vi "Offset Locking- Main v1.0.vi"() -> ()   [LabVIEW 2017]
uses:
  <vilib>/Utility/error.llb/DialogType.ctl
  <vilib>/measure/mamon.llb/Waveform Peak Detection for 1 Chan.vi
  <vilib>/addons/control/pid/pid.llb/PID Advanced (DBL).vi
  <vilib>/measure/NI_MAPro.lvlib
  <vilib>/addons/control/pid/NI_PID_pid.lvlib
  <vilib>/Analysis/NI_AALBase.lvlib
panel:
  out "Run Time (min)":dbl
  out "standard deviation":dbl format="%0.3e"
  in  "Ref Peak 2":i32=1
  in  "Ref Peak":i32=2
  in  "First Cal Peak":i32
  in  "Last Cal Peak":i32=2
  out "# found":i32
  out "Offset":dbl(graph)
  in  "Manual PZT Control":dbl format="%#_g V"
  in  "Engage PZT PID?":bool
  out "Offset (GHz)":dbl format="%#_4g"
  in  "# of Shots for Averaging":i32=100
  in  "Name Convention":string="Chirp Offset Lock Log"
  in  "Save Directory":path=path "C:/Users/LabUser/Google Drive/Measurements/04-2018"
  out "Four peaks?":bool
  out "PID Output":dbl(graph)
  in  "PID Gains":T1={"proportional gain (Kc)"=-1.0, "integral time (Ti, min)"=0.01, "derivative time (Td, min)"=0.0} {"derivative time (Td, min)" format="%.3f"; "integral time (Ti, min)" format="%.3f"; "proportional gain (Kc)" format="%.3f"}
  in  "Setpoint Range (GHz)":cluster{"setpoint high":dbl, "setpoint low":dbl}={"setpoint high"=7.7901, "setpoint low"=7.7899} {"setpoint high" format="%.4f"; "setpoint low" format="%.4f"}
  out "dt out (s)":dbl format="%.3f"
  in  "Frequency Offset Setpoint (GHz)":dbl=7.79 format="%.3f"
  out "GHz/sec":dbl
  out "dt":dbl format="%#_4g"
  out "Locations":dbl[](array[numeric]) format="%.2p"
  out "Amplitudes":dbl[](array[numeric]) format="%.2p"
  out "2nd Derivatives":dbl[](array[numeric]) format="%.2p"
  out "10 GHz FPI":dynamicdata(graph)
  in  "Stop":bool
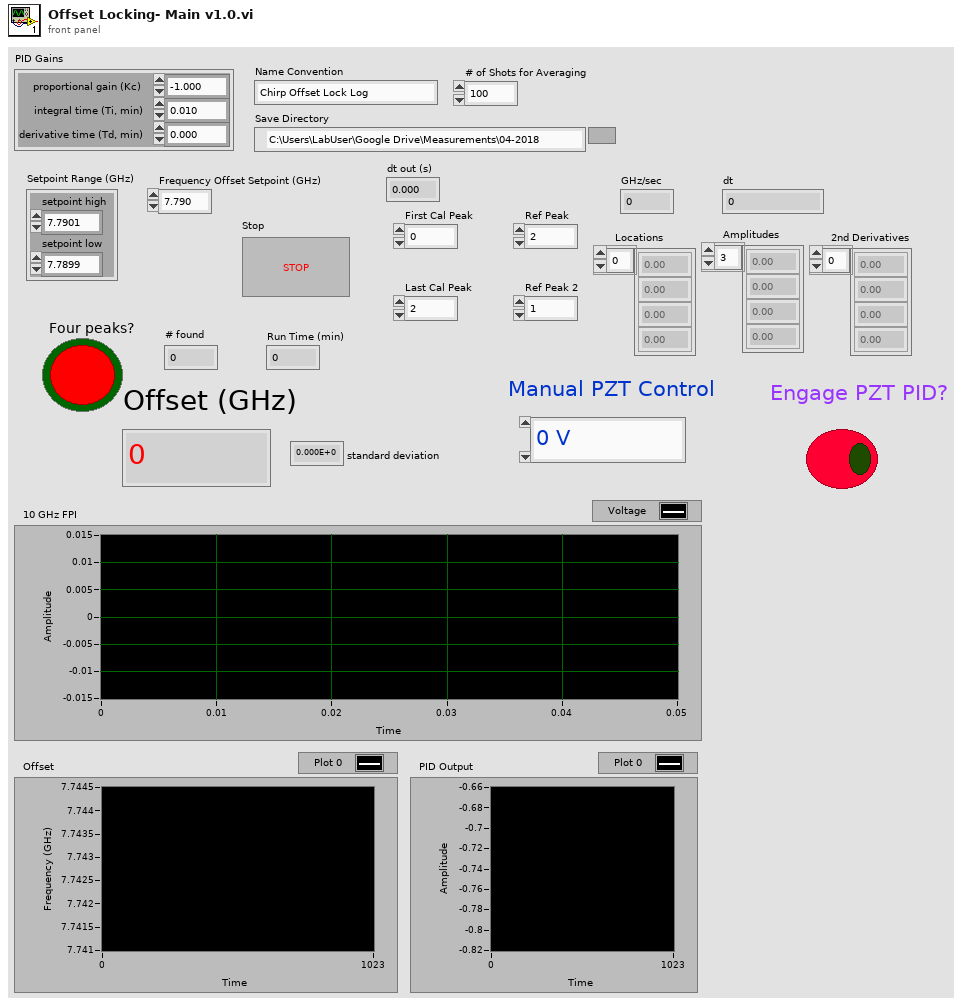
[diagram p1: front panel]
types:
  T1 = cluster{"proportional gain (Kc)":dbl, "integral time (Ti, min)":dbl, "derivative time (Td, min)":dbl}
  T2 = enum8{"Enabled", "Disabled", "Disabled and Grayed Out"}
  T3 = typedef "DialogType.ctl" = u16
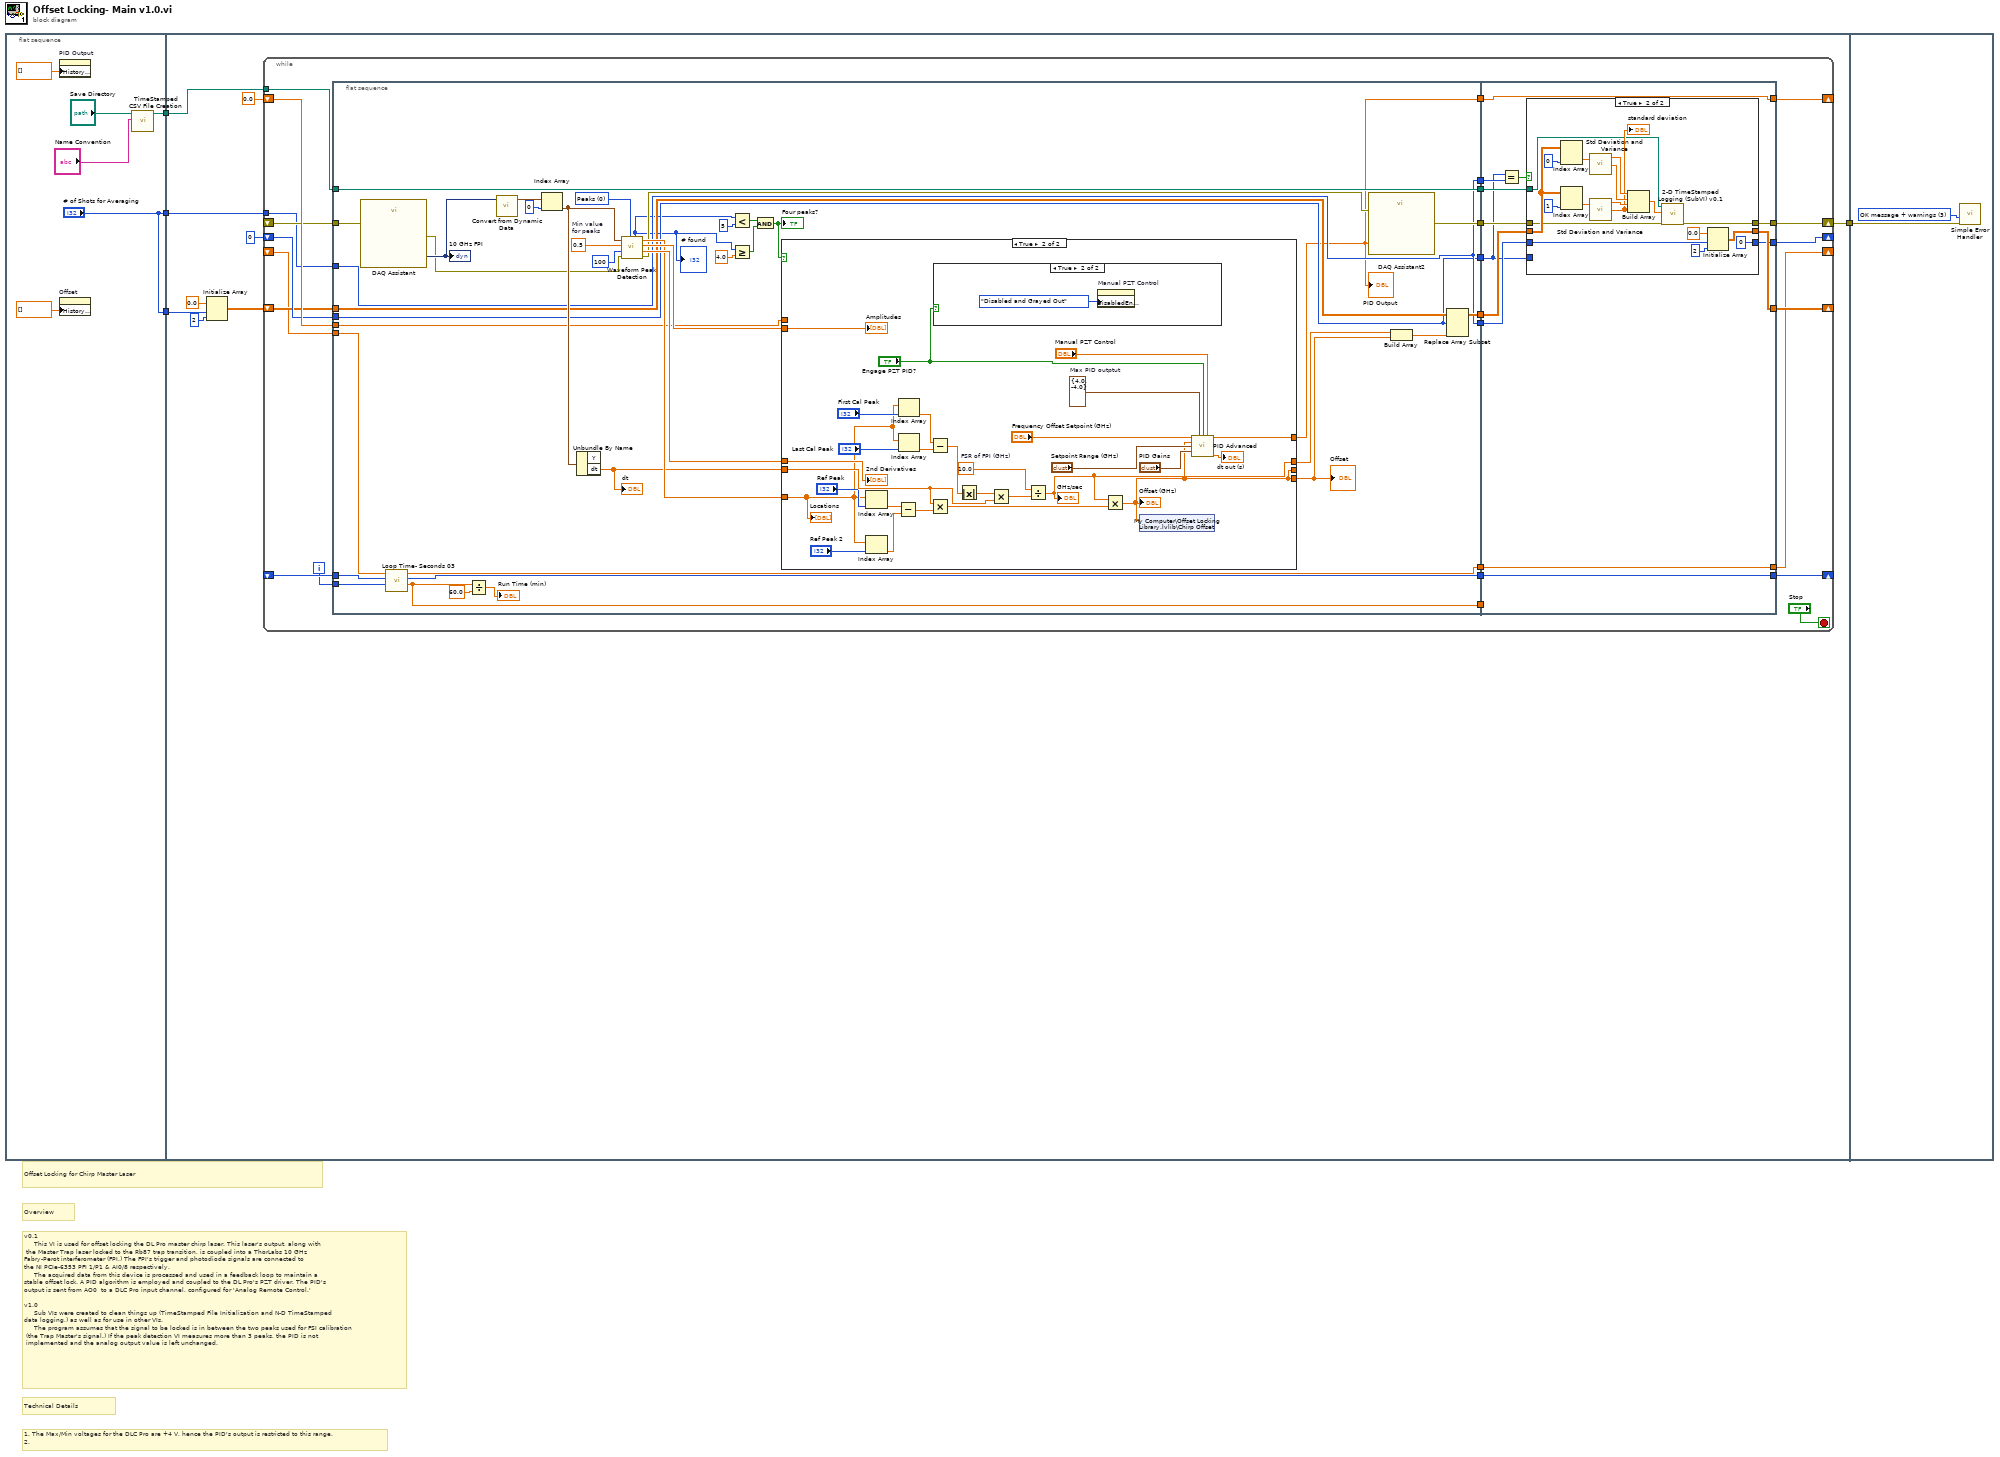
[diagram p0: block diagram]
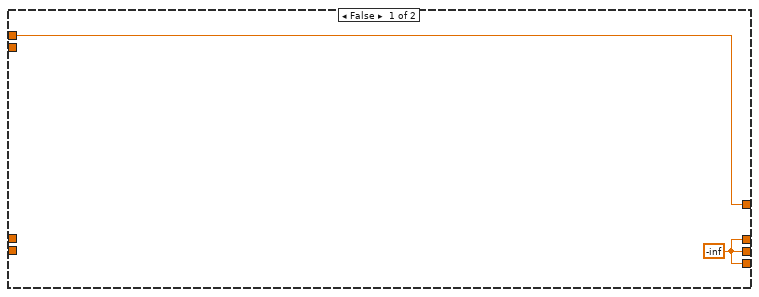
[diagram p2: hidden frame]
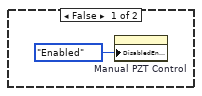
[diagram p3: hidden frame]
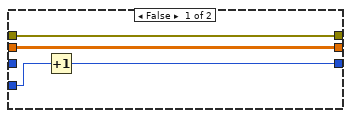
[diagram p4: hidden frame]
diagram:
  # "1. The Max/Min voltages for the DLC Pro are +4 V, hence the PID's output is restricted to this range.\n2."
  # "Technical Details"
  # "v0.1\n     This VI is used for offset locking the DL Pro master chirp laser. This laser's output, along with\n the Master Trap laser locked to the Rb87 trap transition, is coupled into a ThorLabs 10 GHz \nFabry-Perot interferometer (FPI.) The FPI's trigger and photodiode signals are connected to \nthe NI PCIe-6353 PFI 1/P1 & AI0/8 respectively. \n     The acquired data from this device is processed and used in a feedback loop to maintain a \nstable offset lock. A PID algorithm is employed and coupled to the DL Pro's PZT driver. The PID's\noutput is sent from AO0  to a DLC Pro input channel, configured for 'Analog Remote Control.'\n\nv1.0\n     Sub VIs were created to clean things up (TimeStamped File Initialization and N-D TimeStamped \ndata logging,) as well as for use in other VIs.\n     The program assumes that the signal to be locked is in between the two peaks used for FSI calibration\n (the Trap Master's signal.) If the peak detection VI measures more than 3 peaks, the PID is not\n implemented and the analog output value is left unchanged."
  # "Overview"
  # "Offset Locking for Chirp Master Laser"
  n1 = flat-sequence {
    tunnel: [w8] -> w4
    tunnel: ["# of Shots for Averaging"] -> w2
    tunnel: ["# of Shots for Averaging"] -> w1
    tunnel: w4 -> [w18]
    tunnel: [w17] -> w3
    tunnel: w2 -> [w15]
    tunnel: w1 -> [w12]
    tunnel: w3 -> [w152]
    frame #0 {
      n2 = property on="PID Output" class="WFChart (strict)"("History Data"=dbl[] []) -> ()  [unwired: 2 in, 2 out]
      n3 = property on="Offset" class="WFChart (strict)"("History Data"=dbl[] []) -> ()  [unwired: 2 in, 2 out]
      n4 = call "TimeStamped CSV File Creation.vi"("Name Convention"="Name Convention", "Save Directory"="Save Directory") -> ("path"=w8:path)  [unwired: 8 in, 1 out]
    }
    frame #1 {
      n5 = Initialize Array(0.0 ("element"), w12, 2 ("dimension size")) -> (w14:dbl[][])
      n6 = while {
        shift-right: [w38] -> _
        shift-left: 0.0 -> [w44]
        shift-right: [w30] -> w17
        shift-left: _ -> [w43]
        tunnel: w18 -> [w40]
        shift-right: [w28] -> _
        shift-left: 0 -> [w37]
        tunnel: w15 -> [w35]
        shift-right: [w29] -> _
        shift-left: w14 -> [w32]
        shift-right: [w26] -> _
        shift-left: _ -> [w23]
        shift-right: [w24] -> _
        shift-left: _ -> [w22]
        i -> [w21]
        stop <- "Stop" stop-if-true
        n7 = flat-sequence {
          tunnel: w44 -> [w72]
          tunnel: w43 -> [w70]
          tunnel: [w55] -> w42
          tunnel: [w71] -> w41
          tunnel: w40 -> [w67]
          tunnel: [w67] -> w39
          tunnel: w37 -> [w61]
          tunnel: [w61] -> w36
          tunnel: w35 -> [w62]
          tunnel: [w62] -> w34
          tunnel: [w66] -> w33
          tunnel: w32 -> [w65]
          tunnel: [w62] -> w31
          tunnel: [w60] -> w27
          tunnel: [w59] -> w25
          tunnel: w23 -> [w58]
          tunnel: w22 -> [w57]
          tunnel: w21 -> [w56]
          tunnel: [w47] -> w20
          tunnel: w42 -> [w129]
          tunnel: w41 -> [w122]
          tunnel: w39 -> [w123]
          tunnel: [w129] -> w38
          tunnel: w36 -> [w120]
          tunnel: w34 -> [w128]
          tunnel: w33 -> [w125]
          tunnel: w31 -> [w126]
          tunnel: [w124] -> w30
          tunnel: [w121] -> w29
          tunnel: [w119] -> w28
          tunnel: w27 -> [w118]
          tunnel: [w118] -> w26
          tunnel: [w117] -> w24
          tunnel: w25 -> [w117]
          tunnel: w20 -> [_]
          frame #0 {
            w74 = u16 0 items=["Peaks", "Valleys"] ("peaks/valleys")
            w76 = 0.5  # Min value for peaks
            n8 = call "DAQ Assistant"("error in"=w70) -> ("data"=w82:dynamicdata, "error out"=w69:errorcluster)  [unwired: 16 in, 1 out]
            "10 GHz FPI" <- w82
            n9 = call "Loop Time- Seconds 03.vi"("Loop Iteration"=w56, "Shift Registered Time In"=w57, "Shift Registered In"=w58) -> ("t"=w47:dbl, "Shift Registered Time Out"=w59:u32, "Shift Registered Out"=w60:dbl)  [unwired: 6 in]
            n10 = Divide(x=w47, y=60.0) -> (x/y=→"Run Time (min)":dbl)
            n11 = call "Convert from Dynamic Data"("Dynamic Data Type"=w82) -> ("Array of Waveform"=w84:waveform(dbl)[])  [unwired: 3 in]
            n12 = Index Array(array=w84, index=0) -> (element=w79:waveform(dbl))
            n13 = Unbundle By Name(w79) -> ("dt"=w77:dbl)  [unwired: 1 out]
            "dt" <- w77
            n14 = call-poly <vilib>:"Waveform Peak Detection.vi"("peaks/valleys"=w74, "error in"=w69, "width"=100, "threshold"=w76, "Signal In"=w79) -> ("error out"=w68:errorcluster, "2nd Derivatives"=w80:dbl[], "Amplitudes"=w81:dbl[], "Locations"=w78:dbl[], "# found"=w52:i32)  [unwired: 2 in]
            "# found" <- w52
            n15 = Less?(x=w52, y=5) -> (x < y?=w50:bool)
            n16 = Greater Or Equal?(x=w52, y=4.0) -> (x >= y?=w53:bool)
            n17 = And(x=w50, y=w53) -> (x .and. y?=w49:bool)
            "Four peaks?" <- w49
            n18 = case shown="True" w49 {
              tunnel: w81 -> [_ w114]
              tunnel: w80 -> [_ w113]
              tunnel: w78 -> [_ w90]
              tunnel: w77 -> [_ w104]
              tunnel: [w86 w87] -> w55
              tunnel: w72 -> [w86 _]
              tunnel: [w85 w97] -> w64
              tunnel: [w85 w88] -> w54
              tunnel: [w85 w88] -> _
              frame False {
                w85 = -inf
              }
              frame True {
                w98 = cluster{"output high":dbl, "output low":dbl} {"output high"=4.0, "output low"=-4.0}  # Max PID outptut
                w111 = 10.0  # FSR of FPI (GHz)
                n19 = Index Array(array=w90, index="Ref Peak") -> (element=w106:dbl)
                n20 = Index Array(array=w90, index="Ref Peak 2") -> (element=w89:dbl)
                n21 = Subtract(x=w106, y=w89) -> (x-y=w105:dbl)
                n22 = Index Array(array=w90, index="First Cal Peak") -> (element=w107:dbl)
                n23 = Index Array(array=w90, index="Last Cal Peak") -> (element=w112:dbl)
                n24 = Subtract(x=w107, y=w112) -> (x-y=w109:dbl)
                n25 = Multiply(x=w104, y=w105) -> (x*y=w103:dbl)
                n26 = case shown="True" "Engage PZT PID?" {
                  frame False {
                    n27 = property on="Manual PZT Control" class="DigNum (strict)"("DisabledEnum"=T2."Enabled" ("Disabled")) -> ()  [unwired: 2 in, 2 out]
                  }
                  frame True {
                    n28 = property on="Manual PZT Control" class="DigNum (strict)"("DisabledEnum"=T2."Disabled and Grayed Out" ("Disabled")) -> ()  [unwired: 2 in, 2 out]
                  }
                }
                n29 = Absolute Value(x=w109) -> (abs(x)=w108:dbl)
                n30 = Multiply(x=w108, y=w104) -> (x*y=w110:dbl)
                n31 = Divide(x=w111, y=w110) -> (x/y=w97:dbl)
                "GHz/sec" <- w97
                n32 = Multiply(x=w97, y=w103) -> (x*y=w88:dbl)
                "Offset (GHz)" <- w88
                n33 = shared-variable "My Computer\\Offset Locking Library.lvlib\\Chirp Offset"(w88) -> ()  [unwired: 1 in, 1 out]
                n34 = call-poly <vilib>:"PID Advanced.vi"("setpoint"="Frequency Offset Setpoint (GHz)", "output range"=w98, "auto? (T)"="Engage PZT PID?", "manual control"="Manual PZT Control", "process variable"=w88, "setpoint range"="Setpoint Range (GHz)", "PID gains"="PID Gains") -> ("output"=w87:dbl, "dt out (s)"=→"dt out (s)":dbl)  [unwired: 7 in]
                "2nd Derivatives" <- w113
                "Amplitudes" <- w114
                "Locations" <- w90
              }
            }
            "Offset" <- w54
            "PID Output" <- w55
            n35 = call "DAQ Assistant2"("data"=w55, "error in"=w68) -> ("error out"=w71:errorcluster)  [unwired: 16 in, 1 out]
            n36 = Build Array(w64, w54) -> (w63:dbl[])
            n37 = Replace Array Subset(array=w65, new element=w63, index (row)=w61) -> (w66:dbl[][])  [unwired: 1 in]
          }
          frame #1 {
            n38 = Equal?(x=w120, y=w128) -> (x = y?=w127:bool)
            n39 = case shown="True" w127 {
              tunnel: w126 -> [_ w136]
              tunnel: w125 -> [w132 w147]
              tunnel: [w133 w142] -> w124
              tunnel: w123 -> [_ w140]
              tunnel: w122 -> [w133 w139]
              tunnel: [w132 w135] -> w121
              tunnel: w120 -> [w131 _]
              tunnel: [w130 0] -> w119
              frame False {
                n40 = Increment(x=w131) -> (x+1=w130:i32)
              }
              frame True {
                n41 = Index Array(array=w147, index (col)=0 ("disabled index (col)")) -> (element=w150:dbl[])  [unwired: 1 in]
                n42 = Index Array(array=w147, index (col)=1 ("disabled index (col)")) -> (element=w148:dbl[])  [unwired: 1 in]
                n43 = call <vilib>:"Std Deviation and Variance.vi"("X"=w150) -> ("mean"=w146:dbl, "standard deviation"=w145:dbl)  [unwired: 1 in, 1 out]
                n44 = call <vilib>:"Std Deviation and Variance.vi"("X"=w148) -> ("mean"=w144:dbl, "standard deviation"=w143:dbl)  [unwired: 1 in, 1 out]
                "standard deviation" <- w143
                n45 = Build Array(w146, w145, w144, w143) -> (w141:dbl[])
                n46 = call "2-D TimeStamped Logging (SubVI) v0.1.vi"("error in (no error)"=w139, "array"=w141, "path"=w140) -> ("error out"=w142:errorcluster)  [unwired: 8 in]
                n47 = Initialize Array(0.0 ("element"), w136, 2 ("dimension size")) -> (w135:dbl[][])
              }
            }
          }
        }
      }
    }
    frame #2 {
      w153 = T3 3 items=["no dialog", "OK message", "continue or stop message", "OK message + warnings", "continue/stop + warnings"] ("type of dialog (OK msg:1)")
      n48 = call <vilib>:"Simple Error Handler.vi"("type of dialog (OK msg:1)"=w153, "error in (no error)"=w152) -> ()  [unwired: 3 in, 5 out]
    }
  }
